vi "SimAHarduino.vi"() -> ()   [LabVIEW 2019]
uses:
  <vilib>/Simulation/Scripting/Companion Diagram/SimConfigNode/SimParams.ctl
  <vilib>/Simulation/Scripting/Companion Diagram/SimConfigNode/_simSolvers.ctl
  <vilib>/Simulation/Implementation/Shared/SIMSCR Execution Mode.ctl
  <vilib>/Simulation/Param Hierarchy/Typedefs/SIMPH Param Control Actions.ctl
  <vilib>/DAQmx/read.llb/DAQmx Read (Analog DBL 1Chan 1Samp).vi
  <vilib>/Simulation/Implementation/Shared/NILVSim_ParamChanged.vi
  <vilib>/Simulation/Implementation/Shared/NILVSIM_BeginStep.vi
  <vilib>/Simulation/Implementation/Shared/NILVSim_Manager.vi
  <vilib>/Utility/error.llb/Clear Errors.vi
  <vilib>/Simulation/Implementation/Shared/NILVSim_FinalizeModel.vi
  <vilib>/DAQmx/miscellaneous.llb/DAQmx Fill In Error Info.vi
  <vilib>/Simulation/Implementation/Shared/SIM Unbundle Sim Info.vi
  <vilib>/Simulation/Implementation/Shared/NILVSim_Initialize.vi
  <vilib>/Simulation/Utility/Implementation/NILVSim Get Time and IsAcceptedStep.vi
  <vilib>/Simulation/Implementation/Shared/SIMSH Read Queue.vi
  <vilib>/Simulation/Implementation/Shared/NILVSim_GetModelError.vi
  <vilib>/Simulation/Implementation/Shared/SIM Bundle Sim Info.vi
  <vilib>/Simulation/Implementation/XNodeFramework/SimXNode/SimX.xnode
  Air Heater - LabVIEW/Air Heater Black Box Model.vi
  <vilib>/Simulation/Scripting/Companion Diagram/SimConfigNode/SimDog.xnode
  <vilib>/Simulation/Implementation/Shared/NI_SIM_Implementation.lvlib
panel:
  out "Control Chart":dbl(graph)
  out "temp_sp":dbl
  out "u_out":dbl
  out "control signal [u]":dbl
  out "Temperature Chart":cluster{"Tout [1-5V]":dbl, "Setpoint":dbl}(graph)
  in  "Setpoint":dbl(slide) scale=20.0..50.0
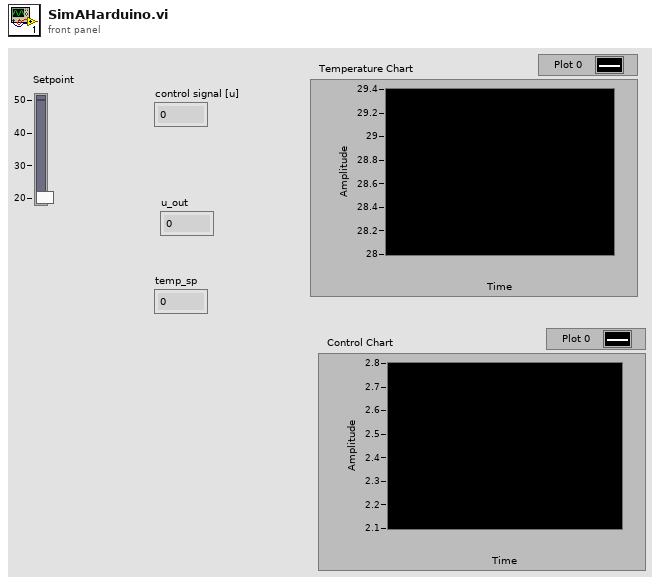
[diagram p1: front panel]
types:
  T1 = enum16{"Simulate to Completion", "Single Time-Step Simulation (Fixed Step Only)"}
  T2 = typedef "SIMSCR Execution Mode.ctl" = enum16{"Simulate to Completion", "Single Time-Step Simulation (Fixed Step Only)"}
  T3 = typedef "SIMPH Param Control Actions.ctl" = enum16{"get params", "set params"}
  T4 = cluster{"SIMSH Sim Time":dbl, "Select":cluster{"s? t:f":dbl}, "Linear Scaling with Points.vi":cluster{"y":dbl}, "Summation 3":cluster{"Result":dbl}, "Square Root":cluster{"sqrt(x)":dbl}, "Gaussian White Noise PtByPt.vi":cluster{"Gaussian white noise":dbl}, "Integrator":cluster{"output":dbl}, "Multiplication":cluster{"Result":dbl}, "Summation":cluster{"Result":dbl}, "Multiplication 2":cluster{"Result":dbl}, "Transport Delay":cluster{"output":dbl}, "Summation 2":cluster{"Result":dbl}}
  T5 = typedef "SimParams.ctl" = cluster{"Initial Time (s)":dbl, "Final Time (s)":dbl, "Step Size (s)":dbl, "ODE Solver":T6, "Minimum Step Size (s)":dbl, "Maximum Step Size (s)":dbl, "Relative Tolerance":dbl, "Absolute Tolerance":dbl, "Software Timing":bool, "Initial Step Size (s)":dbl, "Automatic Fixed Step Size?":bool, "Automatic Discrete Step Size?":bool, "Discrete Step Size (s)":dbl, "Calculate using Time Step":bool, "Solver Wired?":bool, "Prev.Frm.Expected End":u64, "Prev.Frm.Actual End":u64, "Prev.Frm.Finished Late?":bool, "Prev.Iter.Expected End":u64, "Prev.Iter.Actual End":u64, "Prev.Iter.Finished Late?":bool, "Expected Iteration Start":u64, "Actual Iteration Start":u64, "Expected Frame Start":u64, "Actual Frame Start":u64, "Source Name":string, "Name":string, "Period":i64, "Deadline":i64, "Offset":i64, "Start":i64, "Priority":i32, "Timeout":i32, "Processor":i32, "Mode":enum32{"No Change", "Process missed periods, maintain original phase", "Discard missed periods, maintain original phase", "Process missed periods, ignore original phase", "Discard missed periods, ignore original phase"}, "Wakeup reason":enum32{"Normal", "Aborted", "Asynchronous wakeup", "Timing source error", "Timed loop error", "Timeout"}, "Error":errorcluster, "Source Type":string, "Secondary Source Type":string, "Global End Time":u64, "Global Start Time":u64, "Full Solver Reset":bool, "Execution Mode":T2, "Nan/Inf Check":bool, "Custom Solver Library":string, "Solver Is Variable":bool, "custom solver name":string, "Signal Collection Decimation":u32}
  T6 = typedef "_simSolvers.ctl" = enum16{"Runge-Kutta 1 (Euler)", "Runge-Kutta 2", "Runge-Kutta 3", "Runge-Kutta 4", "Runge-Kutta 23 (variable)", "Runge-Kutta 45 (variable)", "BDF (variable)", "Adams-Moulton (variable)", "Rosenbrock (variable)", "Discrete States Only", "SDIRK 4 (variable)", "Radau 5 (variable)", "Radau 9 (variable)", "Radau 13 (variable)", "Radau [Variable Order] (variable)", "Gear's Method (variable)", "Linearizer", "State Query", "Trim Eval", "Custom Solver"}
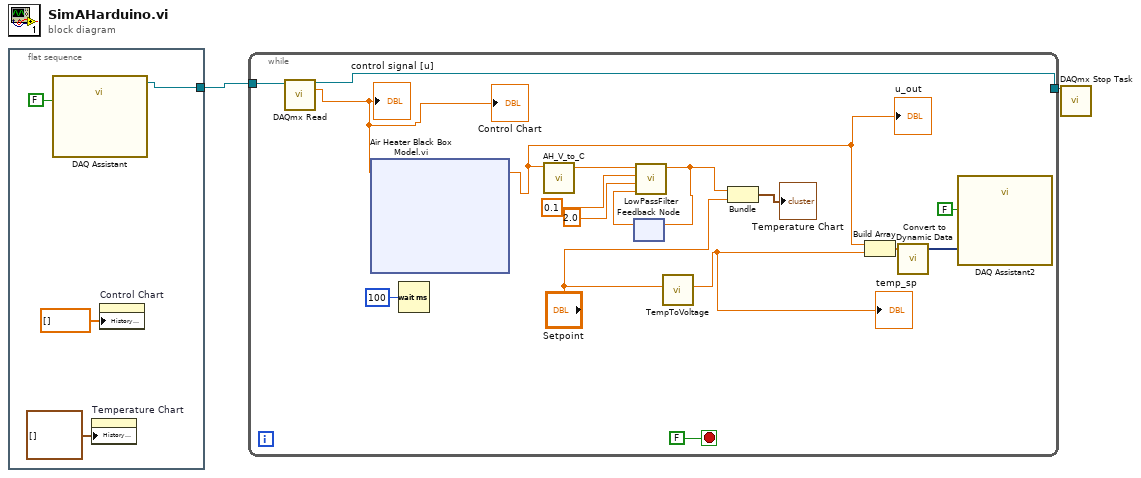
[diagram p0: block diagram]
diagram:
  n1 = flat-sequence {
    tunnel: [w5] -> w2
    frame #0 {
      n2 = call "DAQ Assistant"("stop (T)"=FALSE) -> ("task out"=w5:refnum<k21>)  [unwired: 16 in, 2 out]
      n3 = property on="Temperature Chart" class="WFChart (strict)"("History Data"=cluster{"Tout [1-5V]":dbl, "Setpoint":dbl}[] []) -> ()  [unwired: 2 in, 2 out]
      n4 = property on="Control Chart" class="WFChart (strict)"("History Data"=dbl[] []) -> ()  [unwired: 2 in, 2 out]
    }
  }
  n5 = while {
    tunnel: w2 -> [w19]
    tunnel: [w18] -> w1
    stop <- FALSE stop-if-true
    n6 = call-poly <vilib>:"DAQmx Read.vi"("task/channels in"=w19) -> ("task out"=w18:refnum<k21>, "data"=w7:dbl)  [unwired: 12 in, 1 out]
    "control signal [u]" <- w7
    "Control Chart" <- w7
    n7 = xnode "Air Heater Black Box Model.vi"("Control Signal [0-5V]"=w7) -> ("Tout [1-5V]"=w13:dbl)  [unwired: 2 in, 1 out]
    "u_out" <- w13
    n8 = Wait (ms)(milliseconds to wait=u32 100) -> ()  [unwired: 1 out]
    n9 = call "AH_V_to_C.vi"("Vin[1-5V]"=w13) -> ("Tout[C]"=w12:dbl)  [unwired: 10 in]
    n10 = feedback #1() -> (w11:dbl)  [unwired: 1 in]
    n11 = call "LowPassFilter.vi"("input variable"=w11, "Tf[s]"=2.0, "Ts[s]"=0.1, "u_k"=w12) -> ("output variable"=w10:dbl)  [unwired: 7 in]
    n12 = feedback-in #1(w10) -> ()
    n13 = call "TempToVoltage.vi"("T_out"="Setpoint") -> ("u_out"=w14:dbl)  [unwired: 10 in]
    "temp_sp" <- w14
    n14 = Bundle("output variable"=w10, "Setpoint"="Setpoint") -> (→"Temperature Chart":cluster{"output variable":dbl, "Setpoint":dbl})  [unwired: 1 in]
    n15 = Build Array(w13, w14) -> (w15:dbl[])
    n16 = call "Convert to Dynamic Data"("Array"=w15) -> ("Dynamic Data Type"=w16:dynamicdata)  [unwired: 3 in]
    n17 = call "DAQ Assistant2"("data"=w16, "stop (T)"=FALSE) -> ()  [unwired: 16 in, 2 out]
  }
  n18 = call <vilib>:"DAQmx Stop Task.vi"("task/channels in"=w1) -> ()  [unwired: 13 in, 2 out]
